vi "runcount.vi"(1 "Serial Number":string, 2 "-1?":bool) -> (0 "4th run?":bool)   [LabVIEW 2013]
uses:
  Controls/FailedTests.ctl
  <vilib>/Utility/config.llb/NI_LVConfig.lvlib
  <vilib>/Utility/config.llb/Write Key (I32).vi
  <vilib>/Utility/config.llb/Read Key (I32).vi
panel:
  out "Error Out":errorcluster
  in  "Error In":errorcluster
  out "Unit failed 3x Tests":bool
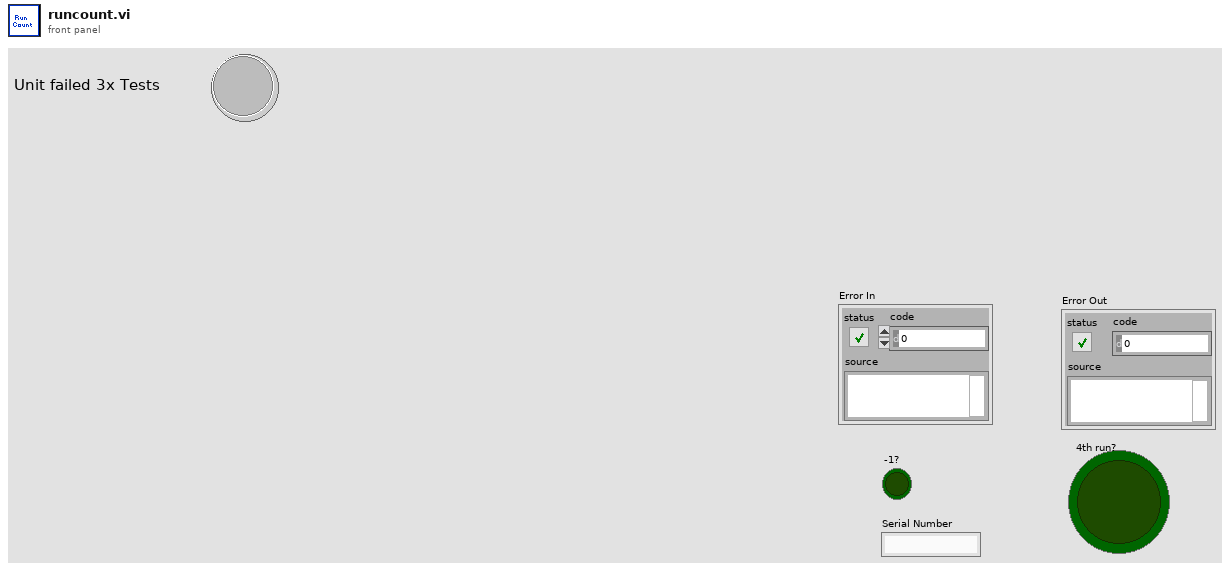
[diagram p1: front panel]
types:
  T1 = typedef "FailedTests.ctl" = enum16{"Initialize", "Add Serial", "Get Serial", "Remove Serial", "Close Config File"}
  T2 = typedef "NI_LVConfig.lvlib/Config Data RefNum.ctl" = refnum<k1>
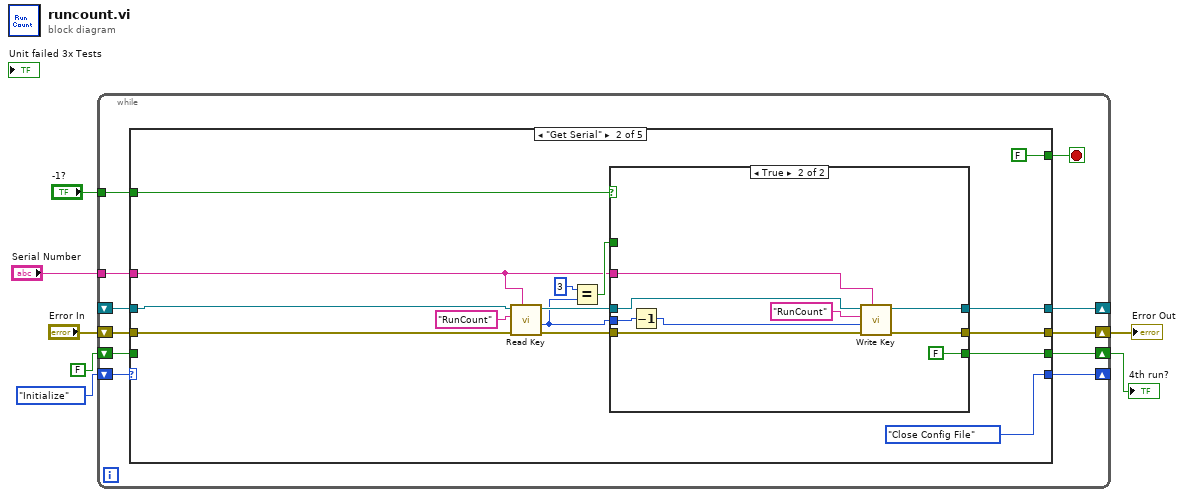
[diagram p0: block diagram]
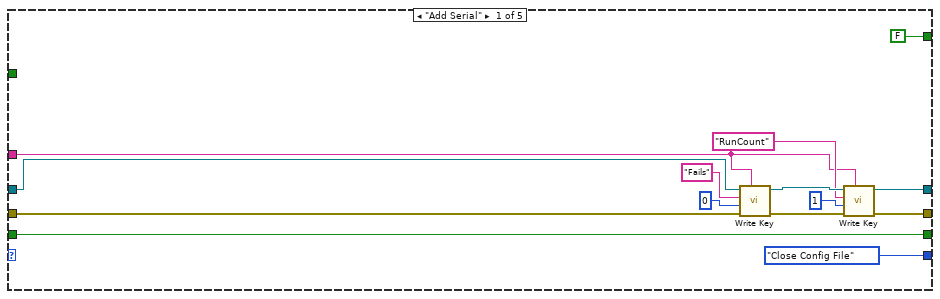
[diagram p2: hidden frame]
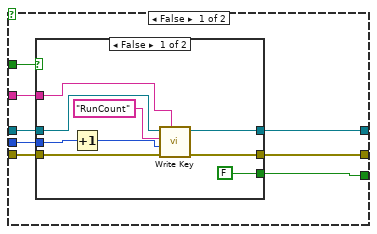
[diagram p3: hidden frame]
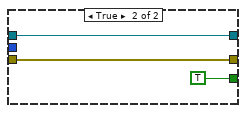
[diagram p4: hidden frame]
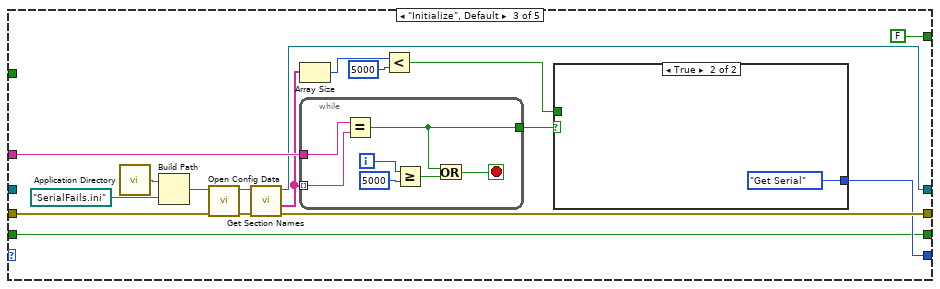
[diagram p5: hidden frame]
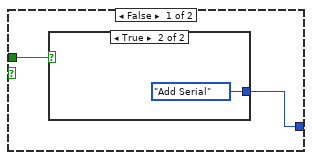
[diagram p6: hidden frame]
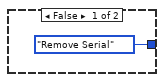
[diagram p7: hidden frame]
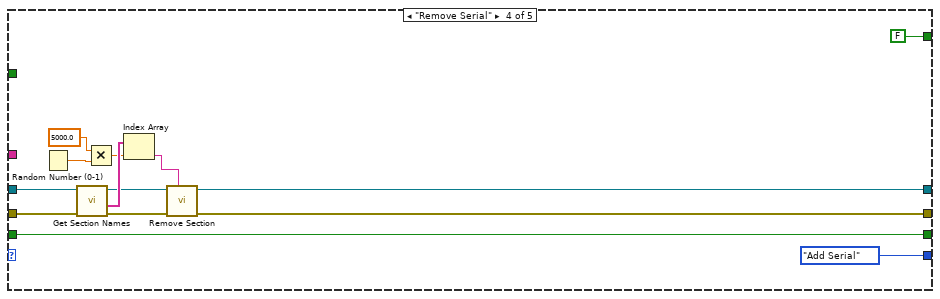
[diagram p8: hidden frame]
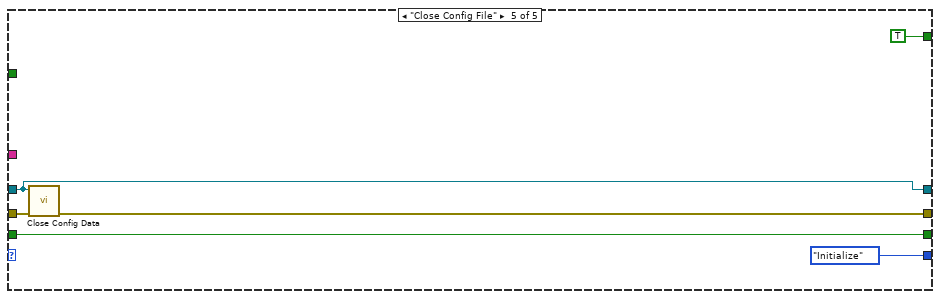
[diagram p9: hidden frame]
diagram:
  n1 = while {
    shift-right: [w13] -> _
    shift-left: FailedTests."Initialize" -> [w18]
    shift-right: [w15] -> w6
    shift-left: "Error In" -> [w17]
    shift-right: [w16] -> _
    shift-left: _ -> [w12]
    tunnel: "Serial Number" -> [w14]
    shift-right: [w10] -> w3
    shift-left: FALSE ("4th run?") -> [w9]
    tunnel: "-1?" -> [w8]
    stop <- w11 stop-if-true
    n2 = case shown="\"Get Serial\"" w18 {
      tunnel: w17 -> [w31 w46 w93 w118 w125]
      tunnel: [w25 w39 w82 w108 w121] -> w16
      tunnel: [w21 w38 w90 w109 w124] -> w15
      tunnel: w14 -> [w20 w40 w89 _ _]
      tunnel: [FailedTests."Close Config File" FailedTests."Close Config File" w84 FailedTests."Add Serial" FailedTests."Initialize"] -> w13
      tunnel: w12 -> [w32 w47 _ w119 w121]
      tunnel: [FALSE FALSE FALSE FALSE TRUE] -> w11
      tunnel: [w19 w34 w77 w106 w120] -> w10
      tunnel: w9 -> [w19 _ w77 w106 w120]
      tunnel: w8 -> [_ w33 _ _ _]
      frame "Add Serial" {
        n3 = call-poly <vilib>:"Write Key.vi"("section"=w20, "error in (no error)"=w31, "value"=0, "key"="Fails", "refnum"=w32) -> ("error out"=w22:errorcluster, "refnum out"=w26:T2)  [unwired: 4 in, 1 out]
        n4 = call-poly <vilib>:"Write Key.vi"("section"=w20, "error in (no error)"=w22, "value"=1, "key"="RunCount", "refnum"=w26) -> ("error out"=w21:errorcluster, "refnum out"=w25:T2)  [unwired: 4 in, 1 out]
      }
      frame "Get Serial" {
        n5 = call-poly <vilib>:"Read Key.vi"("section"=w40, "error in (no error)"=w46, "key"="RunCount", "refnum"=w47) -> ("error out"=w41:errorcluster, "value"=w37:i32, "refnum out"=w42:T2)  [unwired: 4 in, 1 out]
        n6 = Equal?(x=3, y=w37) -> (x = y?=w43:bool)
        n7 = case shown="True" w33 {
          tunnel: w43 -> [w55 _]
          tunnel: w42 -> [w54 w70]
          tunnel: w41 -> [w53 w73]
          tunnel: w40 -> [w52 w74]
          tunnel: [w51 w69] -> w39
          tunnel: [w50 w72] -> w38
          tunnel: w37 -> [w49 w68]
          tunnel: [w48 FALSE ("4th run?")] -> w34
          frame False {
            n8 = case shown="False" w55 {
              tunnel: w54 -> [w64 w65]
              tunnel: w53 -> [w63 w66]
              tunnel: w52 -> [w59 _]
              tunnel: [w58 w65] -> w51
              tunnel: [w57 w66] -> w50
              tunnel: w49 -> [w62 _]
              tunnel: [FALSE ("4th run?") TRUE ("4th run?")] -> w48
              frame False {
                n9 = Increment(x=w62) -> (x+1=w61:i32)
                n10 = call-poly <vilib>:"Write Key.vi"("section"=w59, "error in (no error)"=w63, "value"=w61, "key"="RunCount", "refnum"=w64) -> ("error out"=w57:errorcluster, "refnum out"=w58:T2)  [unwired: 4 in, 1 out]
              }
              frame True {
              }
            }
          }
          frame True {
            n11 = Decrement(x=w68) -> (x-1=w76:i32)
            n12 = call-poly <vilib>:"Write Key.vi"("section"=w74, "error in (no error)"=w73, "value"=w76, "key"="RunCount", "refnum"=w70) -> ("error out"=w72:errorcluster, "refnum out"=w69:T2)  [unwired: 4 in, 1 out]
          }
        }
      }
      frame "Initialize", Default {
        n13 = call <vilib>:"Application Directory.vi"() -> ("Application Directory"=w81:path)
        n14 = Build Path(base path=w81, name or relative path=path "SerialFails.ini") -> (appended path=w79:path)
        n15 = call <vilib>:"Open Config Data.vi"("error in (no error)"=w93, "configuration file path"=w79) -> ("error out"=w91:errorcluster, "refnum"=w92:T2)  [unwired: 7 in, 1 out]
        n16 = call <vilib>:"Get Section Names.vi"("error in (no error)"=w91, "refnum"=w92) -> ("error out"=w90:errorcluster, "section names"=w88:string[], "refnum out"=w82:T2)  [unwired: 7 in]
        n17 = Array Size(array=w88) -> (size(s)=w87:i32)
        n18 = while {
          tunnel: w88 -> [w105] mode=indexing
          tunnel: w89 -> [w104]
          tunnel: [w100] -> w85
          i -> [w103]
          stop <- w101 stop-if-true
          n19 = Equal?(x=w104, y=w105) -> (x = y?=w100:bool)
          n20 = Greater Or Equal?(x=w103, y=5000) -> (x >= y?=w99:bool)
          n21 = Or(x=w100, y=w99) -> (x .or. y?=w101:bool)
        }
        n22 = Less?(x=w87, y=5000) -> (x < y?=w83:bool)
        n23 = case shown="True" w85 {
          tunnel: [w94 FailedTests."Get Serial"] -> w84
          tunnel: w83 -> [w95 _]
          frame False {
            n24 = case shown="True" w95 {
              tunnel: [FailedTests."Remove Serial" FailedTests."Add Serial"] -> w94
              frame False {
              }
              frame True {
              }
            }
          }
          frame True {
          }
        }
      }
      frame "Remove Serial" {
        n25 = Random Number (0-1)() -> (number: 0 to 1=w115:dbl)
        n26 = call <vilib>:"Get Section Names.vi"("error in (no error)"=w118, "refnum"=w119) -> ("error out"=w111:errorcluster, "section names"=w116:string[], "refnum out"=w112:T2)  [unwired: 7 in]
        n27 = Multiply(x=5000.0, y=w115) -> (x*y=w113:dbl)
        n28 = Index Array(array=w116, index=w113) -> (element=w110:string)
        n29 = call <vilib>:"Remove Section.vi"("section"=w110, "error in (no error)"=w111, "refnum"=w112) -> ("error out"=w109:errorcluster, "refnum out"=w108:T2)  [unwired: 6 in, 1 out]
      }
      frame "Close Config File" {
        n30 = call <vilib>:"Close Config Data.vi"("error in (no error)"=w125, "refnum"=w121) -> ("error out"=w124:errorcluster)  [unwired: 8 in, 1 out]
      }
    }
  }
  "Error Out" <- w6
  "4th run?" <- w3
